vi "software_timestamp.vi"(6 "timeout (25000ms)":i32=25000, 8 "error in (no error)":errorcluster, 11 "daemon reference in":refnum<k5>) -> (0 "error out":errorcluster, 2 "response":string, 3 "daemon reference out":refnum<k5>, 5 "command out":string="software_timestamp")   [LabVIEW 2017]
doc: "<b>Command: </b>\"software_timestamp\"\n\n<b>Description: </b> Queries the target for the software timestamp.\n\n<b>Parameters: </b> None\n____________________________________________\nDIPC 692 Daemon API 10.0.0.1\nSam Tee - Dyson Technology Ltd\nCopyright (c) 2024, Dyson Technology Ltd"
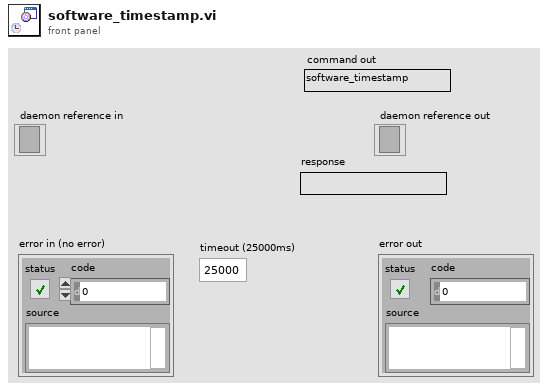
[diagram p1: front panel]
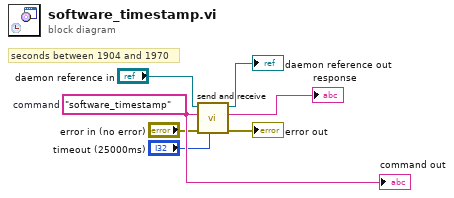
[diagram p0: block diagram]
diagram:
  w5 = "software_timestamp"  # command
  # "seconds between 1904 and 1970"
  n1 = call "send and receive.vi"("timeout (25000ms)"="timeout (25000ms)", "error in (no error)"="error in (no error)", "command"=w5, "daemon reference in"="daemon reference in") -> ("error out"=→"error out":errorcluster, "response"=→"response":string, "daemon reference out"=→"daemon reference out":refnum<k5>)  [unwired: 5 in]
  "command out" <- w5
